vi "niRFUtil MT UTIL Kaiser-Bessel Interp FIR design.vi"(2 "Stop Attenuation":dbl format="%.2f", 3 "interpolation factor":i32=1) -> (1 "h":T1 min=0 max=127 format="%.2f")   [LabVIEW 2015, in "niRFUtil.lvlib"]
uses:
  niRFUtil.lvlib
  Includes/niRFUtil INC Real Array.ctl
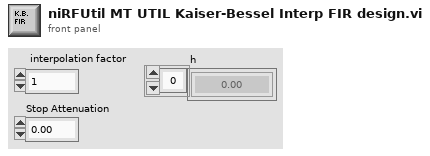
[diagram p1: front panel]
types:
  T1 = typedef "niRFUtil.lvlib/niRFUtil INC Real Array.ctl" = sgl[]
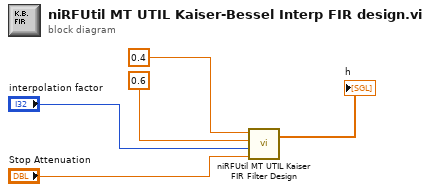
[diagram p0: block diagram]
diagram:
  n1 = call "niRFUtil MT UTIL Kaiser FIR Filter Design.vi"("Stop Attenuation"="Stop Attenuation", "sampling freq: fs"="interpolation factor", "high cutoff freq: fh"=0.6, "low cutoff freq: fl"=0.4) -> ("h"=→"h":dbl[])  [unwired: 1 out]
